vi "Read All Keys and Values.vi"(8 "error in":errorcluster, 11 "LVJSON.lvlib:JSON Object.lvclass":refnum<class "JSON Object.lvclass">) -> (0 "error out":errorcluster, 1 "values":refnum<class "JSON Datatype.lvclass">[](array[class]), 2 "keys":string[](array[string]))   [LabVIEW 2017, in "LVJSON.lvlib" / "JSON Object.lvclass"]
uses:
  JSON Object.lvclass
  JSON Datatype/JSON Datatype.lvclass
  JSON Object.lvclass/JSON Object.ctl
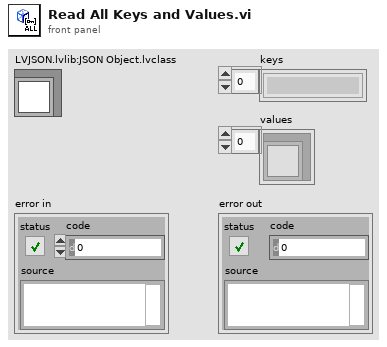
[diagram p1: front panel]
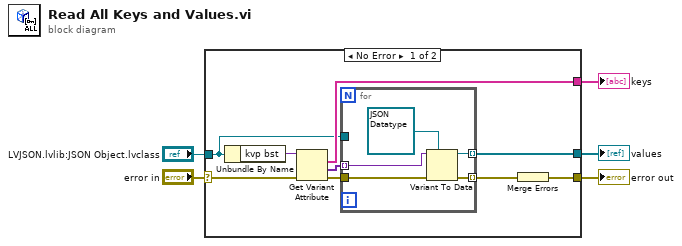
[diagram p0: block diagram]
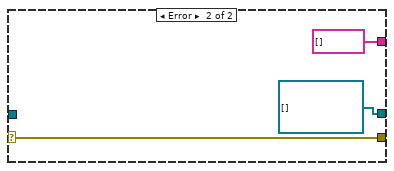
[diagram p2: hidden frame]
diagram:
  n1 = case shown="No Error" "error in" {
    selector: "error in" -> [w10 w22]
    tunnel: [w12 string[] []] -> w5
    tunnel: [w11 refnum<class "JSON Datatype.lvclass">[] []] -> w4
    tunnel: [w8 w22] -> w2
    tunnel: "LVJSON.lvlib:JSON Object.lvclass" -> [w9 _]
    frame No Error {
      n2 = Unbundle By Name(w9) -> ("kvp bst"=w14:variant)
      n3 = Get Variant Attribute(Variant=w14, error in=w10) -> (names=w12:string[], values=w13:variant[], error out=w6:errorcluster)  [unwired: 2 in, 1 out]
      n4 = for {
        tunnel: w9 -> [_]
        tunnel: w13 -> [w18] mode=indexing
        tunnel: [w17] -> w11 mode=indexing
        tunnel: [w16] -> w7 mode=indexing
        tunnel: w6 -> [w15]
        n5 = Variant To Data(error in=w15, type=refnum<class "JSON Datatype.lvclass"> refnum ("JSON Datatype.lvclass"), Variant=w18) -> (data=w17:refnum<class "JSON Datatype.lvclass">, error out=w16:errorcluster)
      }
      n6 = Merge Errors(w7) -> (w8:errorcluster)
    }
    frame Error {
    }
  }
  "keys" <- w5
  "values" <- w4
  "error out" <- w2
